vi "text_message_to_anthropic_message.vi"(1 "message":T2) -> (0 "message out":T1)   [LabVIEW 2020, in "llm_anthropic_chatmodels.lvclass"]
uses:
  llm_anthropic_chatmodels.lvclass
  message_text/message.ctl
  message_text/message_text.lvclass
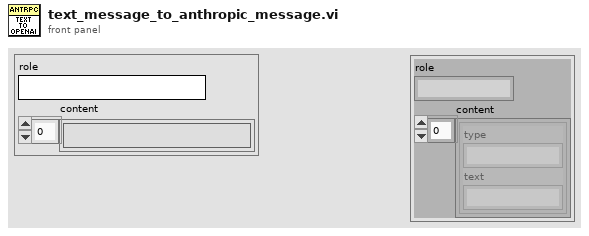
[diagram p1: front panel]
types:
  T1 = cluster{"role":string, "content":cluster{"type":string, "text":string}[]}
  T2 = typedef "message_text.lvclass/message.ctl" = cluster{"role":string, "content":string[]}
  T3 = cluster{"role":string, cluster{"text":string, "text":string}[]}
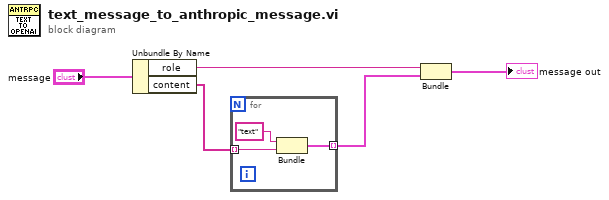
[diagram p0: block diagram]
diagram:
  n1 = Unbundle By Name("message") -> ("role"=w4:string, "content"=w2:string[])
  n2 = for {
    tunnel: w2 -> [w8] mode=indexing
    tunnel: [w6] -> w1 mode=indexing
    n3 = Bundle("text"="text", "text"=w8) -> (w6:cluster{"text":string, "text":string})  [unwired: 1 in]
  }
  n4 = Bundle("role"=w4, w1) -> (→"message out":T3)  [unwired: 1 in]
